vi "Blackjack.vi"() -> ()   [LabVIEW 2013]
panel:
  out "Number of BJs":i32
  out "Percent":dbl
  out "Number of Hands":i32
  out "Hands":string
  in  "Decks":i32
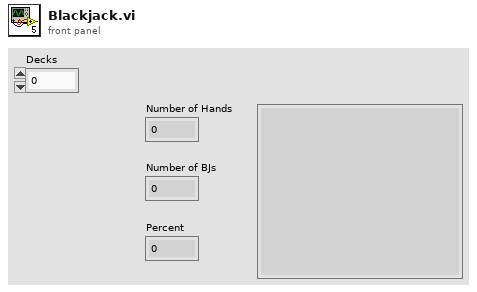
[diagram p1: front panel]
types:
  T1 = cluster{"Pos":dbl, "Value":i32, "Suit":enum16{"Clubs", "Hearts", "Spades", "Diamonds"}}
  T2 = cluster{"Pos":dbl, "Value":i32, "Suit":enum16{"Clubs", "Hearts", "Spades", "Diamonds"}}[]
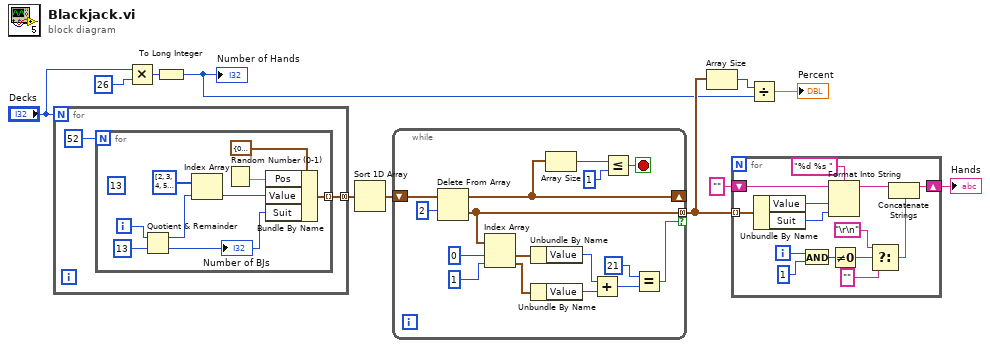
[diagram p0: block diagram]
diagram:
  n1 = for {
    N: "Decks" -> [_]
    tunnel: [w12] -> w11 mode=concatenating
    n2 = for {
      N: 52 -> [_]
      tunnel: [w21] -> w12 mode=indexing
      i -> [w15]
      (unwired) 13 ("y")
      n3 = Quotient & Remainder(x=w15, y=13) -> (x-y*floor(x/y)=w14:i32, floor(x/y)=w16:i32)
      n4 = Index Array(array=i32[] [2, 3, 4, 5, 6, 7, 8, 9, 10, 10, 10, 10, 11], index=w14) -> (element=w17:i32)
      n5 = Random Number (0-1)() -> (number: 0 to 1=w20:dbl)
      n6 = Bundle By Name(cluster=T1 {"Pos"=0.0, "Value"=0, "Suit"=enum."Clubs"} ("Card"), "Pos"=w20, "Value"=w17, "Suit"=w16) -> (w21:T1)
    }
  }
  n7 = Multiply(x="Decks", y=26) -> (x*y=w7:i32)
  n8 = To Long Integer(number=w7) -> (32bit integer=w1:i32)
  "Number of Hands" <- w1
  n9 = Sort 1D Array(array=w11) -> (sorted array=w10:T2)
  n10 = while {
    shift-right: [w36] -> _
    shift-left: w10 -> [w38]
    tunnel: [w27] -> w4 mode=concatenating if=w26
    stop <- w24 stop-if-true
    n11 = Delete From Array(array=w38, length=2) -> (deleted portion=w27:T2, array with subset deleted=w36:T2)  [unwired: 1 in]
    n12 = Index Array(array=w27, index #1=0 ("index"), index #2=1 ("index")) -> (element #1=w33:T1, element #2=w32:T1)
    n13 = Unbundle By Name(w33) -> ("Value"=w30:i32)
    n14 = Unbundle By Name(w32) -> ("Value"=w31:i32)
    n15 = Array Size(array=w36) -> (size(s)=w25:i32)
    n16 = Add(x=w30, y=w31) -> (x+y=w29:i32)
    n17 = Less Or Equal?(x=w25, y=1) -> (x <= y?=w24:bool)
    n18 = Equal?(x=21, y=w29) -> (x = y?=w26:bool)
  }
  n19 = Array Size(array=w4) -> (size(s)=w3:i32)
  n20 = for {
    tunnel: w4 -> [w50] mode=indexing
    shift-right: [w47] -> w8
    shift-left: "" -> [w52]
    i -> [w46]
    n21 = Unbundle By Name(w50) -> ("Value"=w49:i32, "Suit"=w48:enum16{"Clubs", "Hearts", "Spades", "Diamonds"})
    n22 = And(x=w46, y=1) -> (x .and. y?=w44:i32)
    n23 = Format Into String(format string="%d %s ", initial string=w52, w49, w48) -> (resulting string=w51:string)  [unwired: 1 in, 1 out]
    n24 = Not Equal To 0?(x=w44) -> (x != 0?=w43:bool)
    n25 = Select(t="\r\n", s=w43, f="") -> (s? t:f=w40:string)
    n26 = Concatenate Strings(w51, w40) -> (w47:string)
  }
  "Hands" <- w8
  n27 = Divide(x=w3, y=w1) -> (x/y=→"Percent":dbl)
